vi "Configure Channels.vi"(8 "error in (no error)":errorcluster, 11 "Thermometer DAQmx Base CFG in":refnum<class "Thermometer DAQmx Base CFG.lvclass">) -> (0 "error out":errorcluster, 3 "Thermometer DAQmx Base CFG out":refnum<class "Thermometer DAQmx Base CFG.lvclass">)   [LabVIEW 2023, in "Thermometer DAQmx Base CFG.lvclass"]
uses:
  Thermometer DAQmx Base CFG.lvclass
  <vilib>/ErrorRing/Error Ring.xnode
  <vilib>/Utility/error.llb/Error Cluster From Error Code.vi
  <resource>/objmgr/daqmx.rc
  Configuration JSON Base/CFG JSON Base.lvclass
  a898c724-ea1f-46ba-a614-e8ac852e6786.vi
  <vilib>/DAQmx/create/channels.llb/DAQmx Create Channel (AI-Temperature-Thermocouple).vi
panel:
  out "Units":i32(ring)=10325 items=["Deg C"=10143, "Deg F"=10144, "Kelvins"=10325, "Deg R"=10145, "From Custom Scale"=10065]
  out "CJC Source":i32(ring)=10116 items=["Built-In"=10200, "Constant Value"=10116, "Channel"=10113]
  out "Couple Type":i32(ring)=10072 items=["J"=10072, "K"=10073, "N"=10077, "R"=10082, "S"=10085, "T"=10086, "B"=10047, "E"=10055]
  out "AI.AutoZeroMode":i32(ring)=10230 items=["None"=10230, "Once"=10244, "Every Sample"=10164]
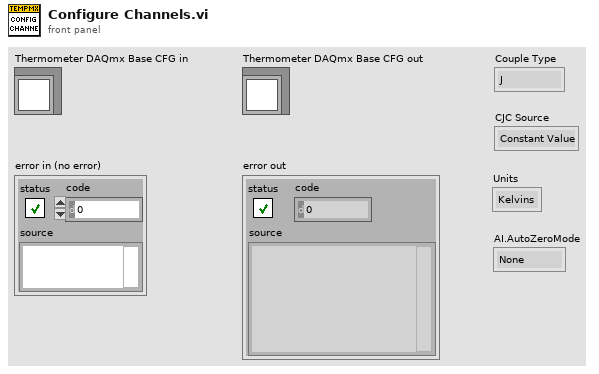
[diagram p1: front panel]
types:
  T1 = cluster{"Name":string, "CJC Source":string, "Max Degree":dbl, "Min Degree":dbl, "CJC Value":dbl, "Thermocouple Type":string, "Units":string, "CJC Channel":string, "Enable Autozero":bool, "Autozero Mode":string}[]
  T2 = typedef "LVStringsAndValuesArrayTypeDef_I32.ctl" = cluster{"String":string, "Value":i32}[]
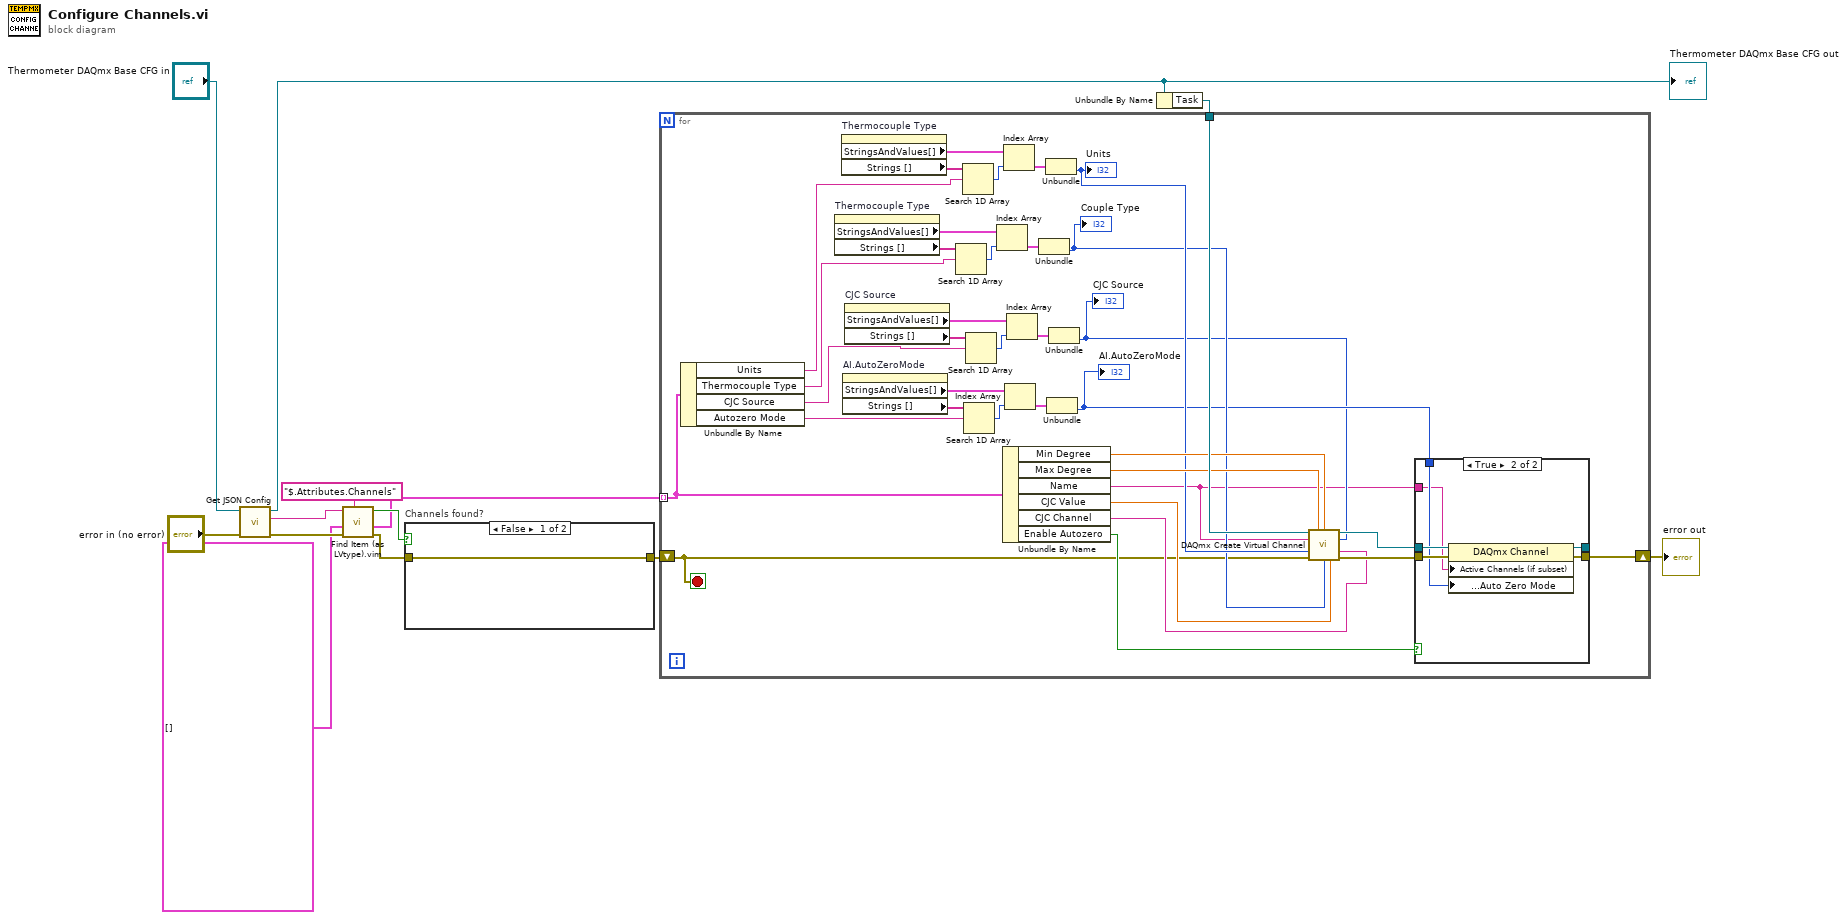
[diagram p0: block diagram]
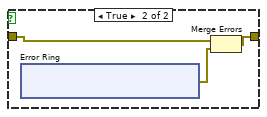
[diagram p3: hidden frame]
diagram:
  n1 = call "Get JSON Config.vi"("error in (no error)"="error in (no error)", "CFG Base in"="Thermometer DAQmx Base CFG in") -> ("error out"=w11:errorcluster, "<JSON>Config>"=w9:string, "CFG Base out"=w1:refnum<class "Thermometer DAQmx Base CFG.lvclass">)  [unwired: 7 in]
  "Thermometer DAQmx Base CFG out" <- w1
  n2 = call "Find Item (as LVtype).vim"("$Path or Item Name"="$.Attributes.Channels", "error in (no error)"=w11, "Data Type and Default Value"=T1 [], "JSON"=w9) -> ("error out"=w7:errorcluster, "Data"=w5:T1, "Found"=w8:bool)  [unwired: 4 in, 1 out]
  n3 = case "Channels found?" shown="False" w8 {
    tunnel: w7 -> [w14 w17]
    tunnel: [w14 w15] -> w6
    frame False {
    }
    frame True {
      n4 = xnode "Error Ring"() -> ("error out"=w16:errorcluster)
      n5 = Merge Errors(w17, w16) -> (w15:errorcluster)
    }
  }
  n6 = Unbundle By Name(w1) -> ("Task"=w3:refnum<k21>)
  n7 = for {
    tunnel: w5 -> [w43] mode=indexing
    tunnel: w3 -> [w42]
    shift-right: [w24] -> w2
    shift-left: w6 -> [w23]
    stop <- w23 stop-if-true
    n8 = Unbundle By Name(w43) -> ("Units"=w35:string, "Thermocouple Type"=w57:string, "CJC Source"=w49:string, "Autozero Mode"=w44:string)
    n9 = property on="Thermocouple Type" class="Ring (strict)"() -> ("StringsAndValues[]"=w56:T2, "Strings []"=w58:string[])  [unwired: 2 in, 2 out]
    n10 = property on="Thermocouple Type" class="Ring (strict)"() -> ("StringsAndValues[]"=w37:T2, "Strings []"=w36:string[])  [unwired: 2 in, 2 out]
    n11 = property on="AI.AutoZeroMode" class="Ring (strict)"() -> ("StringsAndValues[]"=w46:T2, "Strings []"=w45:string[])  [unwired: 2 in, 2 out]
    n12 = property on="CJC Source" class="Ring (strict)"() -> ("StringsAndValues[]"=w52:T2, "Strings []"=w53:string[])  [unwired: 2 in, 2 out]
    n13 = Search 1D Array(1D array=w58, element=w57) -> (index of element=w55:i32)  [unwired: 1 in]
    n14 = Search 1D Array(1D array=w36, element=w35) -> (index of element=w38:i32)  [unwired: 1 in]
    n15 = Search 1D Array(1D array=w45, element=w44) -> (index of element=w47:i32)  [unwired: 1 in]
    n16 = Search 1D Array(1D array=w53, element=w49) -> (index of element=w51:i32)  [unwired: 1 in]
    n17 = Index Array(array=w56, index=w55) -> (element=w54:cluster{"String":string, "Value":i32})
    n18 = Unbundle By Name(w43) -> ("Min Degree"=w40:dbl, "Max Degree"=w41:dbl, "Name"=w25:string, "CJC Value"=w32:dbl, "CJC Channel"=w28:string, "Enable Autozero"=w26:bool)
    n19 = Index Array(array=w37, index=w38) -> (element=w39:cluster{"String":string, "Value":i32})
    n20 = Index Array(array=w46, index=w47) -> (element=w48:cluster{"String":string, "Value":i32})
    n21 = Index Array(array=w52, index=w51) -> (element=w50:cluster{"String":string, "Value":i32})
    n22 = Unbundle(w54) -> ("Value"=w33:i32)  [unwired: 1 out]
    "Couple Type" <- w33
    n23 = Unbundle(w39) -> ("Value"=w34:i32)  [unwired: 1 out]
    "Units" <- w34
    n24 = Unbundle(w48) -> ("Value"=w31:i32)  [unwired: 1 out]
    "AI.AutoZeroMode" <- w31
    n25 = Unbundle(w50) -> ("Value"=w27:i32)  [unwired: 1 out]
    "CJC Source" <- w27
    n26 = call-poly <vilib>:"DAQmx Create Virtual Channel.vi"("task in"=w42, "maximum value"=w41, "minimum value"=w40, "physical channels"=w25, "cjc source"=w27, "units"=w34, "cjc channel"=w28, "error in"=w23, "thermocouple type"=w33, "cjc value"=w32) -> ("task out"=w30:refnum<k21>, "error out"=w29:errorcluster)  [unwired: 4 in]
    n27 = case shown="True" w26 {
      tunnel: w30 -> [w59 w66]
      tunnel: w29 -> [w60 w65]
      tunnel: [w60 w64] -> w24
      tunnel: [w59 w63] -> _
      tunnel: w31 -> [_ w62]
      tunnel: w25 -> [_ w61]
      frame False {
      }
      frame True {
        n28 = property class="DAQmx Channel"(reference=w66, error in=w65, "Active Channels (if subset)"=w61, "Analog Input:General Properties:Advanced:High Accuracy Settings:Auto Zero Mode"=w62) -> (reference out=w63:refnum<k21>, error out=w64:errorcluster)
      }
    }
  }
  "error out" <- w2
